vi "subsriber.vi"() -> ()   [LabVIEW 2022 SP3]
panel:
  in  "stop":bool
  out "Boolean":bool
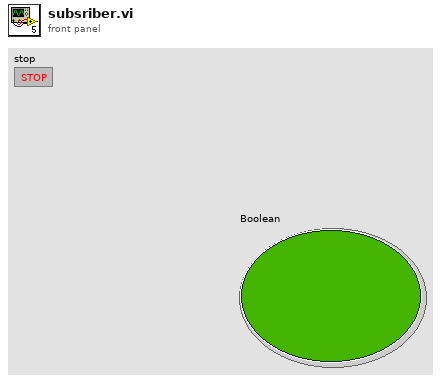
[diagram p1: front panel]
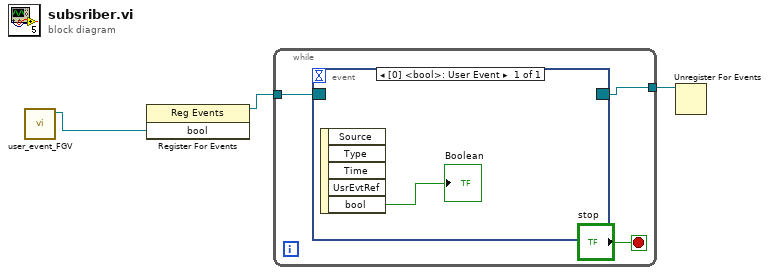
[diagram p0: block diagram]
diagram:
  n1 = call "user_event_FGV.vi"() -> ("bool"=w3:refnum<user-event>)  [unwired: 11 in]
  n2 = register-events(w3) -> (reference out=w2:refnum<event-registration>)  [unwired: 2 in, 1 out]
  n3 = while {
    tunnel: w2 -> [w6]
    tunnel: [w5] -> w1
    stop <- "stop" stop-if-true
    n4 = event shown="[0] <bool>: User Event" {
      selector: w6 -> [_]
      dyn-events: [_] -> w5
      timeout: _ -> [_]
      event User Event {
        n5 = event-data() -> ("bool"=→"Boolean":bool)  [unwired: 1 in, 4 out]
      }
    }
  }
  n6 = Unregister For Events(event registration refnum=w1) -> ()  [unwired: 1 in, 1 out]
